vi "save data.vi"(9 "method":T1={"sampling interval"=0.1, "samples to average"=1, "data interval"=0.0, "stream data"=FALSE, "file path"=refnum, "command"={"command"=enum."Idle", "start time (ms)"=0, "Channel Indices"=[], "Scans per Sample"=1}} {"command"."Scans per Sample" min=1; "data interval" format="%.2f"; "samples to average" min=1 step=1; "sampling interval" format="%.2f"}, 10 "channel strings":string[](array[string]), 11 "voltage data":sgl[][](array[numeric]) format="%.2f") -> ()   [LabVIEW 2010]
uses:
  DAC apps/support/method.ctl
  DataServer/command cluster.ctl
  DataServer/command.ctl
  <vilib>/Utility/file.llb/Write To Spreadsheet File (DBL).vi
panel:
  # "s"
  # "s"
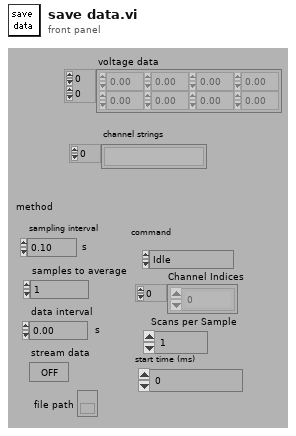
[diagram p1: front panel]
types:
  T1 = typedef "method.ctl" = cluster{"sampling interval":sgl, "samples to average":u32, "data interval":sgl, "stream data":bool, "file path":refnum<file>, "command":T2}
  T2 = typedef "command cluster.ctl" = cluster{"command":T3, "start time (ms)":u32, "Channel Indices":i32[], "Scans per Sample":i32}
  T3 = typedef "command.ctl" = enum16{"Idle", "Send Data", "Send 1 Scan", "Logoff"}
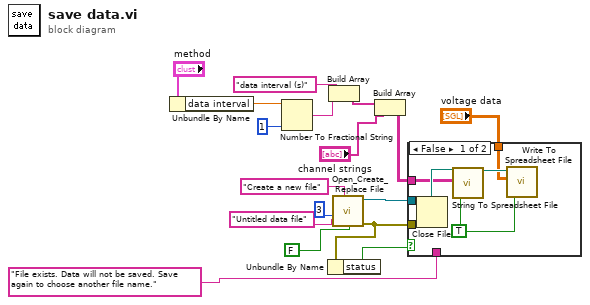
[diagram p0: block diagram]
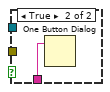
[diagram p2: hidden frame]
diagram:
  n1 = Unbundle By Name("method") -> ("data interval"=w15:sgl)
  n2 = Number To Fractional String(number=w15, precision (6)=1) -> (F-format string=w5:string)  [unwired: 2 in]
  n3 = Build Array("data interval (s)", w5) -> (w6:string[])
  n4 = call <vilib>:"Open_Create_Replace File.vi"("advisory dialog? (display:T)"=FALSE, "default name"="Untitled data file", "prompt"="Create a new file", "function (open:0)"=3) -> ("error out"=w12:errorcluster, "refnum"=w11:refnum<file>)  [unwired: 4 in, 2 out]
  n5 = Unbundle By Name(w12) -> ("status"=w1:bool)
  n6 = Build Array(w6, "channel strings") -> (w7:string[][])
  n7 = case shown="False" w1 {
    tunnel: w12 -> [w24 _]
    tunnel: w11 -> [w22 _]
    tunnel: w7 -> [w21 _]
    tunnel: "File exists. Data will not be saved. Save again to choose another file name." -> [_ w25]
    tunnel: "voltage data" -> [w18 _]
    frame False {
      w20 = TRUE
      n8 = Close File(refnum=w22, error in=w24) -> (path=w23:path)  [unwired: 1 out]
      n9 = call "String To Spreadsheet File.vi"("append to file? (new file:F)"=w20, "2D data"=w21, "file path (dialog if empty)"=w23) -> ("new file path (Not A Path if cancelled)"=w19:path)  [unwired: 5 in]
      n10 = call-poly <vilib>:"Write To Spreadsheet File.vi"("append to file? (new file:F)"=w20, "2D data"=w18, "file path (dialog if empty)"=w19) -> ()  [unwired: 5 in, 1 out]
    }
    frame True {
      n11 = One Button Dialog(message=w25) -> ()  [unwired: 1 in, 1 out]
    }
  }
